vi "updateBall.vi"(8 "error in (no error)":errorcluster, 10 "old Ball":refnum<class "Ball.lvclass">, 11 "Ball in":refnum<class "Ball.lvclass">) -> (0 "error out":errorcluster, 3 "Ball out":refnum<class "Ball.lvclass">)   [LabVIEW 2023, in "Ball.lvclass"]
uses:
  Ball.lvclass
  Object_class/Object.lvclass/Object.ctl
  Ball.lvclass/Ball.ctl
  Object_class/Read x.vi
  Object_class/Read y.vi
  Read v_x.vi
  Read v_y.vi
  Object_class/Read pos_est_x.vi
  Object_class/Read pos_est_y.vi
  Read Valid.vi
  Object_class/Write x.vi
  Object_class/Write y.vi
  Write v_x.vi
  Write v_y.vi
  Object_class/Write pos_est_x.vi
  Object_class/Write pos_est_y.vi
  Write Valid.vi
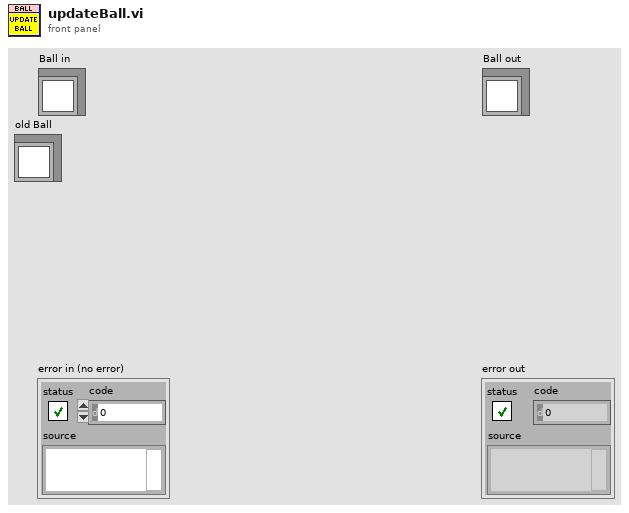
[diagram p1: front panel]
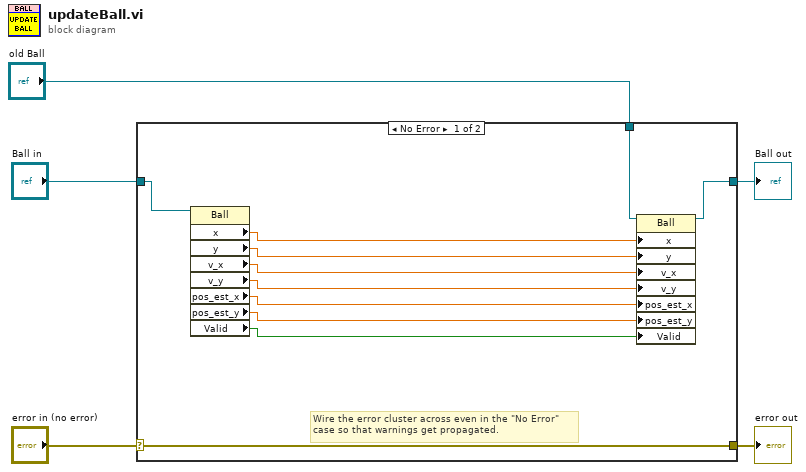
[diagram p0: block diagram]
diagram:
  n1 = case shown="No Error" "error in (no error)" {
    selector: "error in (no error)" -> [w16 w18]
    tunnel: [w16 w18] -> w4
    tunnel: [w14 w17] -> w2
    tunnel: "Ball in" -> [w15 w17]
    tunnel: "old Ball" -> [w13 _]
    frame No Error {
      # "Wire the error cluster across even in the \"No Error\"\ncase so that warnings get propagated."
      n2 = property class="Ball"(reference=w15) -> ("x"=w12:dbl, "y"=w11:dbl, "v_x"=w10:dbl, "v_y"=w9:dbl, "pos_est_x"=w8:dbl, "pos_est_y"=w7:dbl, "Valid"=w6:bool)  [unwired: 1 in, 2 out]
      n3 = property class="Ball"(reference=w13, "x"=w12, "y"=w11, "v_x"=w10, "v_y"=w9, "pos_est_x"=w8, "pos_est_y"=w7, "Valid"=w6) -> (reference out=w14:refnum<class "Ball.lvclass">)  [unwired: 1 in, 1 out]
    }
    frame Error {
    }
  }
  "error out" <- w4
  "Ball out" <- w2
